vi "Get Device Settings.vi"(8 "error in":errorcluster, 11 "EDS in":refnum<class "EDS.lvclass">) -> (0 "error out":errorcluster, 2 "Device Info":string[][](array[string]), 3 "EDS out":refnum<class "EDS.lvclass">)   [LabVIEW 2024]
uses:
  EDS.lvclass
  EDS.lvclass/EDS.ctl
  <vilib>/Utility/config.llb/NI_LVConfig.lvlib
  <vilib>/Utility/config.llb/Read Key (String).vi
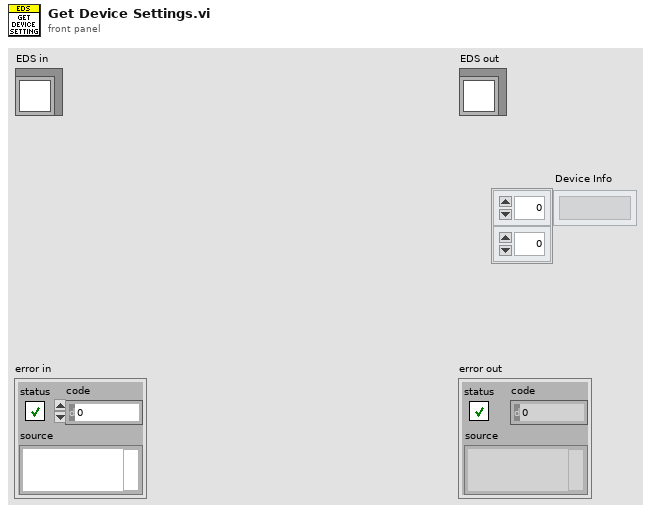
[diagram p1: front panel]
types:
  T1 = typedef "NI_LVConfig.lvlib/Config Data RefNum.ctl" = refnum<k1>
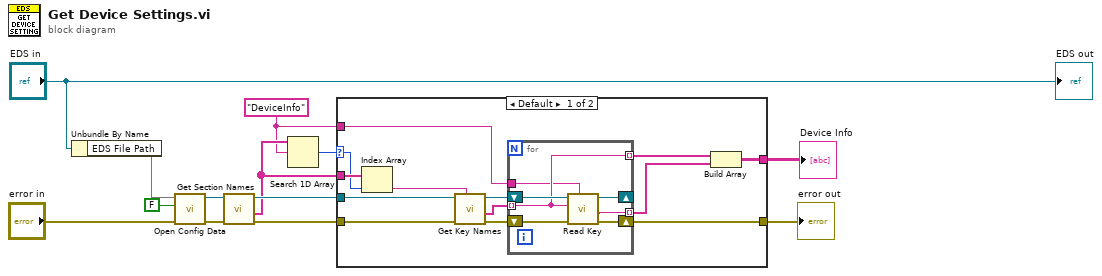
[diagram p0: block diagram]
diagram:
  w5 = "DeviceInfo" ("element")
  n1 = Unbundle By Name("EDS in") -> ("EDS File Path"=w10)
  n2 = call <vilib>:"Open Config Data.vi"("error in (no error)"="error in", "create file if necessary (T)"=FALSE, "configuration file path"=w10) -> ("error out"=w13:errorcluster, "refnum"=w12:T1)  [unwired: 6 in, 1 out]
  n3 = call <vilib>:"Get Section Names.vi"("error in (no error)"=w13, "refnum"=w12) -> ("error out"=w9:errorcluster, "section names"=w6:string[], "refnum out"=w8:T1)  [unwired: 7 in]
  n4 = Search 1D Array(1D array=w6, element=w5) -> (index of element=w7:i32)  [unwired: 1 in]
  n5 = case shown="Default" w7 {
    selector: w7 -> [w20 _]
    tunnel: w9 -> [w26 w34]
    tunnel: w8 -> [w25 _]
    tunnel: w6 -> [w21 _]
    tunnel: w5 -> [w18 _]
    tunnel: [w15 w34] -> w2
    tunnel: [w14 _] -> w1
    frame Default {
      n6 = Index Array(array=w21, index=w20) -> (element=w19:string)
      n7 = call <vilib>:"Get Key Names.vi"("section"=w19, "error in (no error)"=w26, "refnum"=w25) -> ("error out"=w24:errorcluster, "key names"=w22:string[], "refnum out"=w23:T1)  [unwired: 5 in, 1 out]
      n8 = for {
        shift-right: [w29] -> w15
        shift-left: w24 -> [w33]
        tunnel: w22 -> [w28] mode=indexing
        shift-right: [w31] -> _
        shift-left: w23 -> [w32]
        tunnel: [w30] -> w17 mode=indexing
        tunnel: [w28] -> w16 mode=indexing
        tunnel: w18 -> [w27]
        n9 = call-poly <vilib>:"Read Key.vi"("section"=w27, "error in (no error)"=w33, "key"=w28, "refnum"=w32) -> ("error out"=w29:errorcluster, "value"=w30:string, "refnum out"=w31:T1)  [unwired: 4 in, 1 out]
      }
      n10 = Build Array(w16, w17) -> (w14:string[][])
    }
    frame -1 {
    }
  }
  "error out" <- w2
  "Device Info" <- w1
  "EDS out" <- "EDS in"
